vi "TEST Object Manual Bounds (Non Default Scaling Overlapping).vi"() -> ()   [LabVIEW 2021, in "IObject.lvclass"]
uses:
  IObject.lvclass
  <vilib>/Utility/miscctls.llb/LVRectTypeDef.ctl
  Object/Object.lvclass
panel:
  in  "OK Button 4":bool
  in  "OK Button 3":bool
  in  "OK Button 2":bool
  in  "Bounds":T1={"Left"=100, "Top"=50, "Right"=200, "Bottom"=150}
  in  "OK Button 1":bool
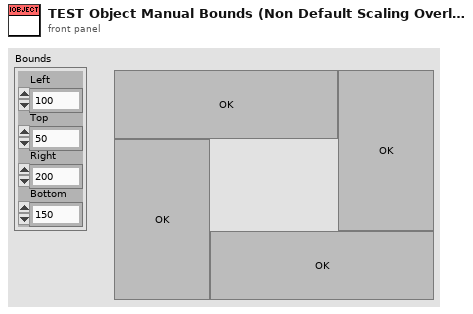
[diagram p1: front panel]
types:
  T1 = typedef "LVRectTypeDef.ctl" = cluster{"Left":i16, "Top":i16, "Right":i16, "Bottom":i16}
  T2 = cluster{"Left":dbl, "Top":dbl, "Right":dbl, "Bottom":dbl}[]
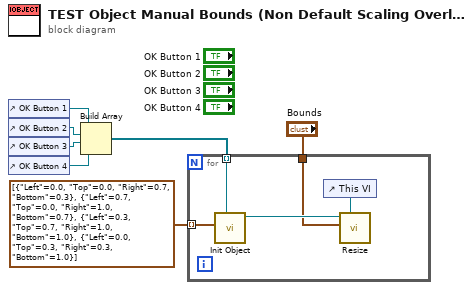
[diagram p0: block diagram]
diagram:
  n1 = control-ref of="OK Button 1"() -> (w7:refnum<vi>)
  n2 = control-ref of="OK Button 2"() -> (w6:refnum<vi>)
  n3 = control-ref of="OK Button 3"() -> (w5:refnum<vi>)
  n4 = control-ref of="OK Button 4"() -> (w4:refnum<vi>)
  n5 = Build Array(w7, w6, w5, w4) -> (w3:refnum<vi>[])
  n6 = for {
    tunnel: T2 [{"Left"=0.0, "Top"=0.0, "Right"=0.7, "Bottom"=0.3}, {"Left"=0.7, "Top"=0.0, "Right"=1.0, "Bottom"=0.7}, {"Left"=0.3, "Top"=0.7, "Right"=1.0, "Bottom"=1.0}, {"Left"=0.0, "Top"=0.3, "Right"=0.3, "Bottom"=1.0}] -> [w10] mode=indexing
    tunnel: w3 -> [w9] mode=indexing
    tunnel: "Bounds" -> [w8]
    n7 = call "Init Object.vi"("GObj Refnum"=w9, "A [0, 0, 1, 1]"=w10) -> ("MMI Scaling out"=w12:refnum<class "Object.lvclass">)  [unwired: 8 in, 1 out]
    n8 = control-ref of="This VI"() -> (w11:refnum<vi>)
    n9 = call-dynamic "Resize.vi"("VI Refnum"=w11, "Bounds"=w8, "MMI Scaling in"=w12) -> ()  [unwired: 6 in, 3 out]
  }
